vi "Process New Channels.vi"(2 "Channel Settings ducktype":T3(array[cluster])=[{"Name"="sim1", "Terminal Information"={"IO Device"=enum."none", "Channel"=0, "Sensor Type"=enum."Voltage"}}, {"Name"="sim2", "Terminal Information"={"IO Device"=enum."none", "Channel"=1, "Sensor Type"=enum."Voltage"}}, {"Name"="sim3", "Terminal Information"={"IO Device"=enum."none", "Channel"=5, "Sensor Type"=enum."Voltage"}}], 3 "Channel Settings in":T4[](array[typedef])=[{"Name"="sim1", "Terminal Information"={"IO Device"=enum."none", "Channel"=0, "Sensor Type"=enum."Voltage"}, "Calibration Information"={"Excitation Voltage"=1.0, "Calibration Factor"=1.0, "Zero Value"=0.0, "Calibration Formula"="", "Units"="V"}}, {"Name"="sim2", "Terminal Information"={"IO Device"=enum."none", "Channel"=1, "Sensor Type"=enum."Voltage"}, "Calibration Information"={"Excitation Voltage"=1.0, "Calibration Factor"=1.0, "Zero Value"=0.0, "Calibration Formula"="", "Units"="V"}}, {"Name"="sim4", "Terminal Information"={"IO Device"=enum."none", "Channel"=-1, "Sensor Type"=enum."Voltage"}, "Calibration Information"={"Excitation Voltage"=1.0, "Calibration Factor"=1.0, "Zero Value"=0.0, "Calibration Formula"="(x-x0) / (Ve * CF)", "Units"="dB"}}]) -> (0 "Channel Settings out":T4[](array[typedef]))   [LabVIEW 2021, in "Settings.lvlib"]
doc: "Update the existing channels in 'Channel Settings in' with the values from 'Channel Settings ducktype', and append any additional channels in the ducktype array."
uses:
  Settings.lvlib
  Acquisition/Channel Settings.ctl
  Acquisition/IO Device.ctl
  Acquisition/Sensor Type.ctl
  Acquisition/Acquisition.lvlib
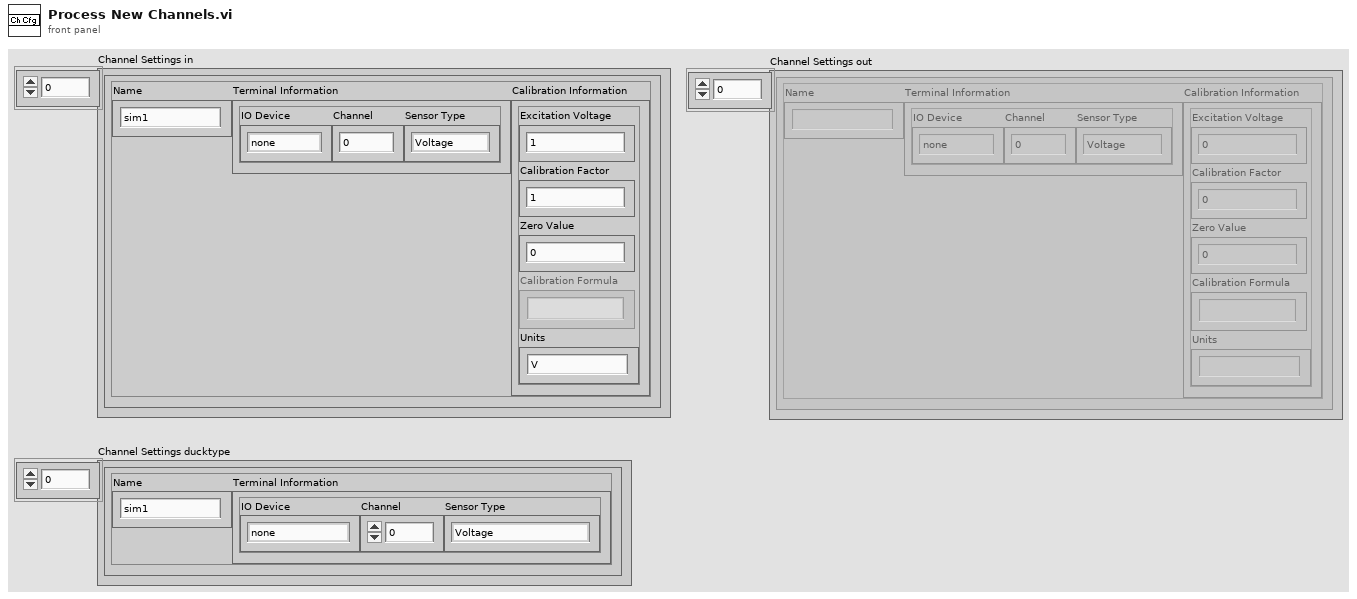
[diagram p1: front panel]
types:
  T1 = typedef "Acquisition.lvlib/IO Device.ctl" = enum16{"none", "9219", "9401"}
  T2 = typedef "Acquisition.lvlib/Sensor Type.ctl" = enum16{"Voltage", "Load", "Pressure", "Encoder"}
  T3 = cluster{"Name":string, "Terminal Information":cluster{"IO Device":T1, "Channel":i32, "Sensor Type":T2}}[]
  T4 = typedef "Acquisition.lvlib/Channel Settings.ctl" = cluster{"Name":string, "Terminal Information":cluster{"IO Device":T1, "Channel":i32, "Sensor Type":T2}, "Calibration Information":cluster{"Excitation Voltage":dbl, "Calibration Factor":dbl, "Zero Value":dbl, "Calibration Formula":string, "Units":string}}
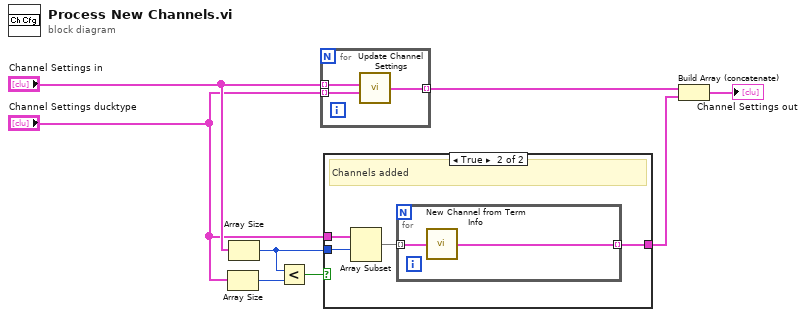
[diagram p0: block diagram]
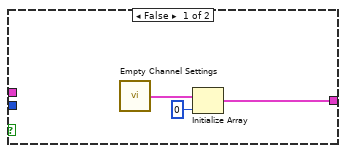
[diagram p2: hidden frame]
diagram:
  n1 = Array Size(array="Channel Settings ducktype") -> (size(s)=w7:i32)
  n2 = Array Size(array="Channel Settings in") -> (size(s)=w4:i32)
  n3 = Less?(x=w4, y=w7) -> (x < y?=w6:bool)
  n4 = for {
    tunnel: "Channel Settings in" -> [w11] mode=indexing
    tunnel: "Channel Settings ducktype" -> [w10] mode=indexing
    tunnel: [w9] -> w3 mode=indexing
    n5 = call "Update Channel Settings.vi"("Channel Settings ducktype"=w10, "Channel Settings in"=w11) -> ("Channel Settings out"=w9:T4)  [unwired: 2 in]
  }
  n6 = case shown="True" w6 {
    tunnel: "Channel Settings ducktype" -> [_ w18]
    tunnel: w4 -> [_ w17]
    tunnel: [w12 w15] -> w2
    frame False {
      n7 = call "Empty Channel Settings.vi"() -> ("Channel Settings"=w13:T4)
      n8 = Initialize Array(w13, 0 ("dimension size")) -> (w12:T4[])
    }
    frame True {
      # "Channels added"
      n9 = Array Subset(array=w18, index=w17) -> (w16:T3)  [unwired: 1 in]
      n10 = for {
        tunnel: w16 -> [w20] mode=indexing
        tunnel: [w19] -> w15 mode=indexing
        n11 = call "New Channel from Term Info.vi"("Channel Settings ducktype"=w20) -> ("New Channel"=w19:T4)
      }
    }
  }
  n12 = Build Array (concatenate)(w3, w2) -> (→"Channel Settings out":T4[])
